vi "Topo & GridSpectr_DriftCorrection_v7.vi"(6 "Internal use":string, 7 "Grid param":T2 {"height (m)" format="%#_6p"; "width (m)" format="%#_6p"; "center Y (m)" format="%#_6p"; "center X (m)" format="%#_6p"}, 8 "Error in (no error)":errorcluster, 9 "Points Y/Index Y":i32, 10 "Points X/Index X":i32, 11 "Method":enum16{"init", "run", "end"}(ring)=enum."end") -> (0 "Error out":errorcluster)   [LabVIEW 2014]
doc: "Example of a measurement VI to be used in the \"Experiments on a Grid\" tool as external VI.\n\nThis example measure the topography and spectroscopy data. The spectroscopy measurements are taken on a subgrid. The data are saved to a sxm and a binary file.\n\n- Nanonis Programming Interface -"
uses:
  <userlib>/Nanonis Prog Interface V5/Nanonis Prog Interface.lvlib
panel:
  in  "max applied Drift Correction":i32=20 min=1 max=100 step=1 format="%.0p"
  in  "Correlate":u16(ring) items=["first Frame", "successive Frames"]
  out "Topo Images taken":i32=14
  in  "Increment":i32=16
  in  "Threshold":i32=3 min=1 step=1
  in  "tip Speed (m/s)":sgl=1e-08 format="%.2p"
  in  "Drift Correction 2":T1
  out "X drift":i32
  out "Y drift":i32
  out "Last Drift detected":i32=40
  in  "MaxImagesBack":i32=40
  in  "Channel index (0-23)":u8=14
  in  "File name":string="single_mol_shortSTS"
  in  "STS Current":dbl=9.999999717180685e-10 format="%#_6p"
  in  "Imaging Current":dbl=5.00000006675716e-11 format="%#_6p"
  in  "zdrift \nDuration (s)":dbl
  in  "Correct z drift":bool
  out "Status":string="finishing"
  in  "Drift correction Pixels":i32=256 caption="Topo Pixels"
  out "Y Offset":dbl format="%#_6p"
  out "X Offset":dbl format="%#_6p"
  out "Points taken":dbl=14.0
  in  "Drift Correction every":i32=16
  in  "Y subgrid spacing":u16=1
  in  "X subgrid spacing":u16=1
  # "GRID points"
  # "Increase this if no Drift was detected for \na certain number of images"
  # "images back"
  # "% of image size"
  # "RUN smart tilt before starting the GRID"
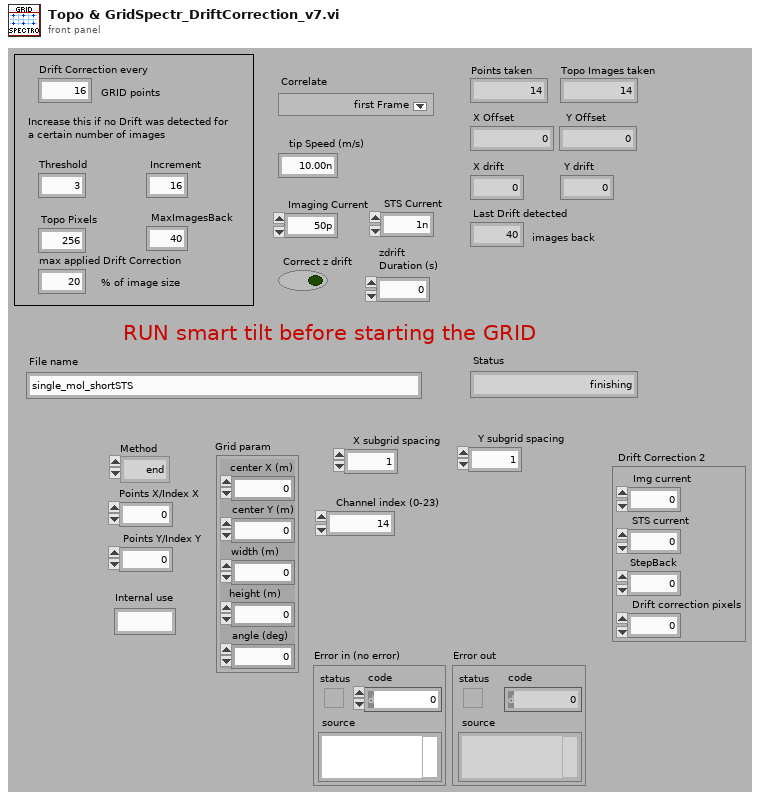
[diagram p1: front panel]
types:
  T1 = cluster{"Img current":dbl, "STS current":dbl, "StepBack":dbl, "Drift correction pixels":dbl}
  T2 = cluster{"center X (m)":sgl, "center Y (m)":sgl, "width (m)":sgl, "height (m)":sgl, "angle (deg)":sgl}
  T3 = cluster{"center X":sgl, "center Y":sgl, "angle":sgl, "width":sgl, "height":sgl, "# pixels":i32, "# lines":i32}
  T4 = cluster{"Name":string, "Calibration":sgl, "Offset":sgl, "Channel index":i32}[]
  T5 = cluster{"up/down":bool, "time/line":sgl, "start time":timestamp, "end time":timestamp}
  T6 = cluster{"Z averaging time (s)":sgl, "Z offset (m)":sgl, "Initial settling time (s)":sgl}
  T7 = cluster{"Max. slew rate (V/s)":sgl, "Settling time (s)":sgl, "Integration time (s)":sgl}
  T8 = cluster{"End settling time (s)":sgl, "Z control time (s)":sgl}
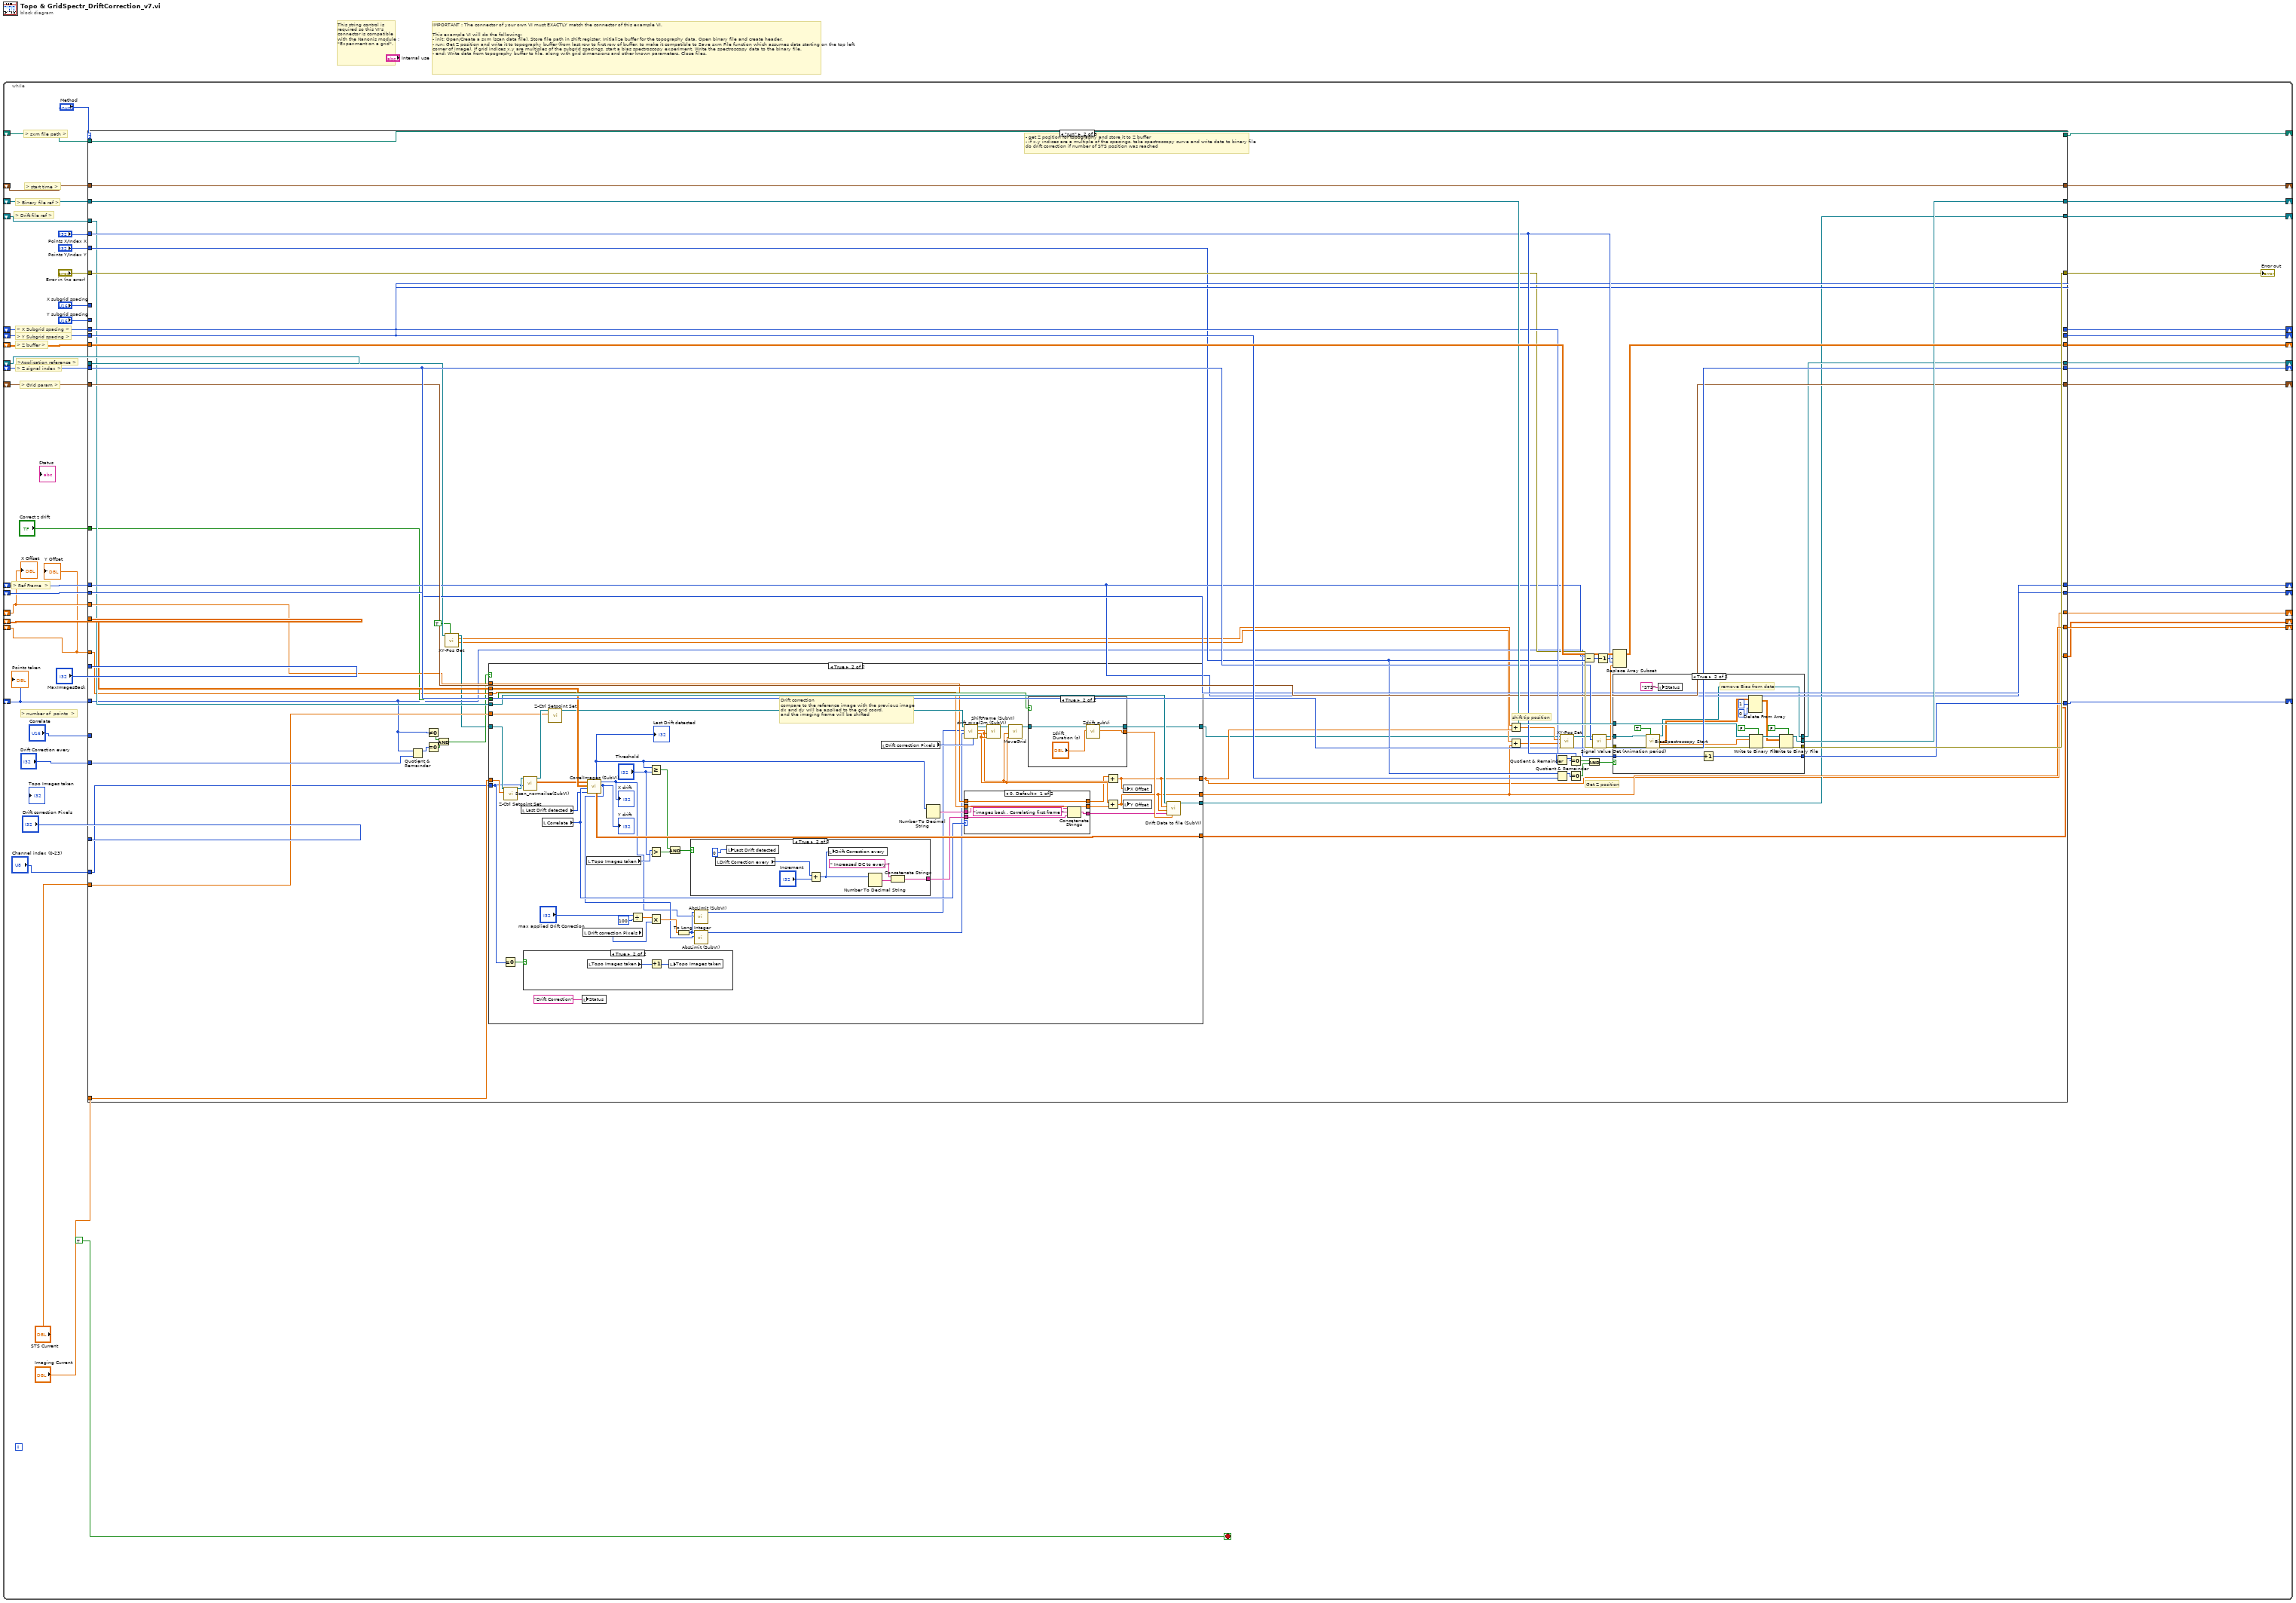
[diagram p0: block diagram]
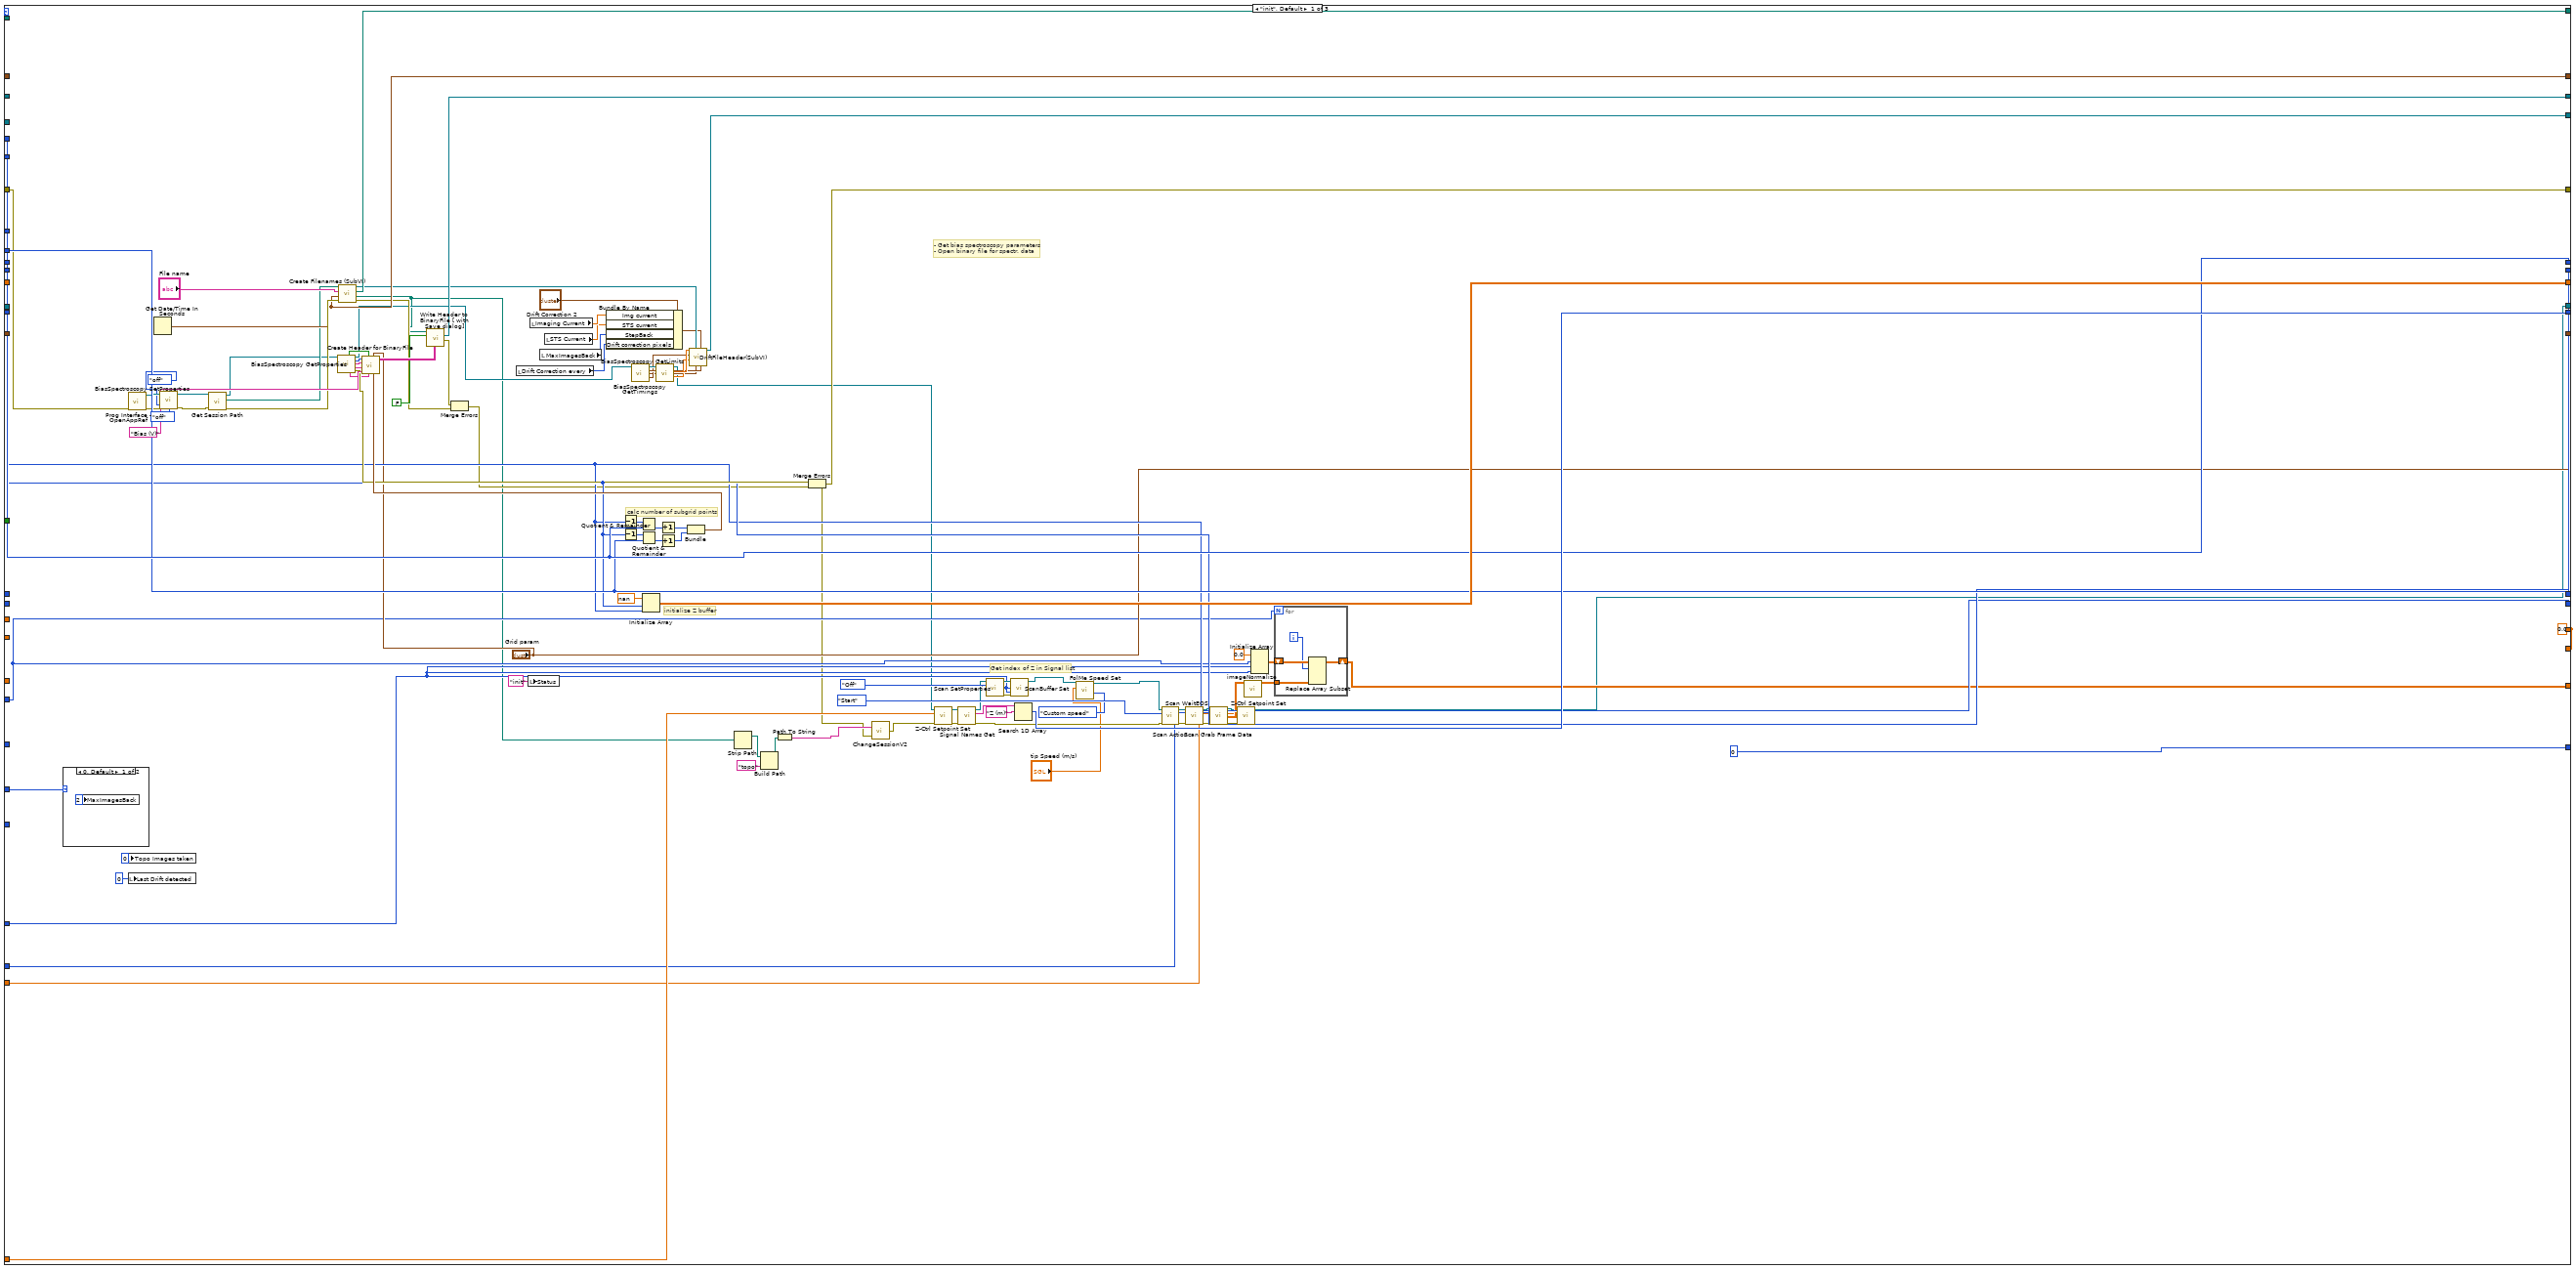
[diagram p2: hidden frame]
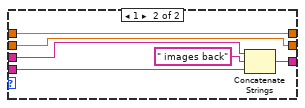
[diagram p5: hidden frame]
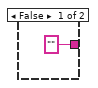
[diagram p7: hidden frame]
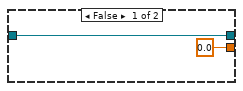
[diagram p8: hidden frame]
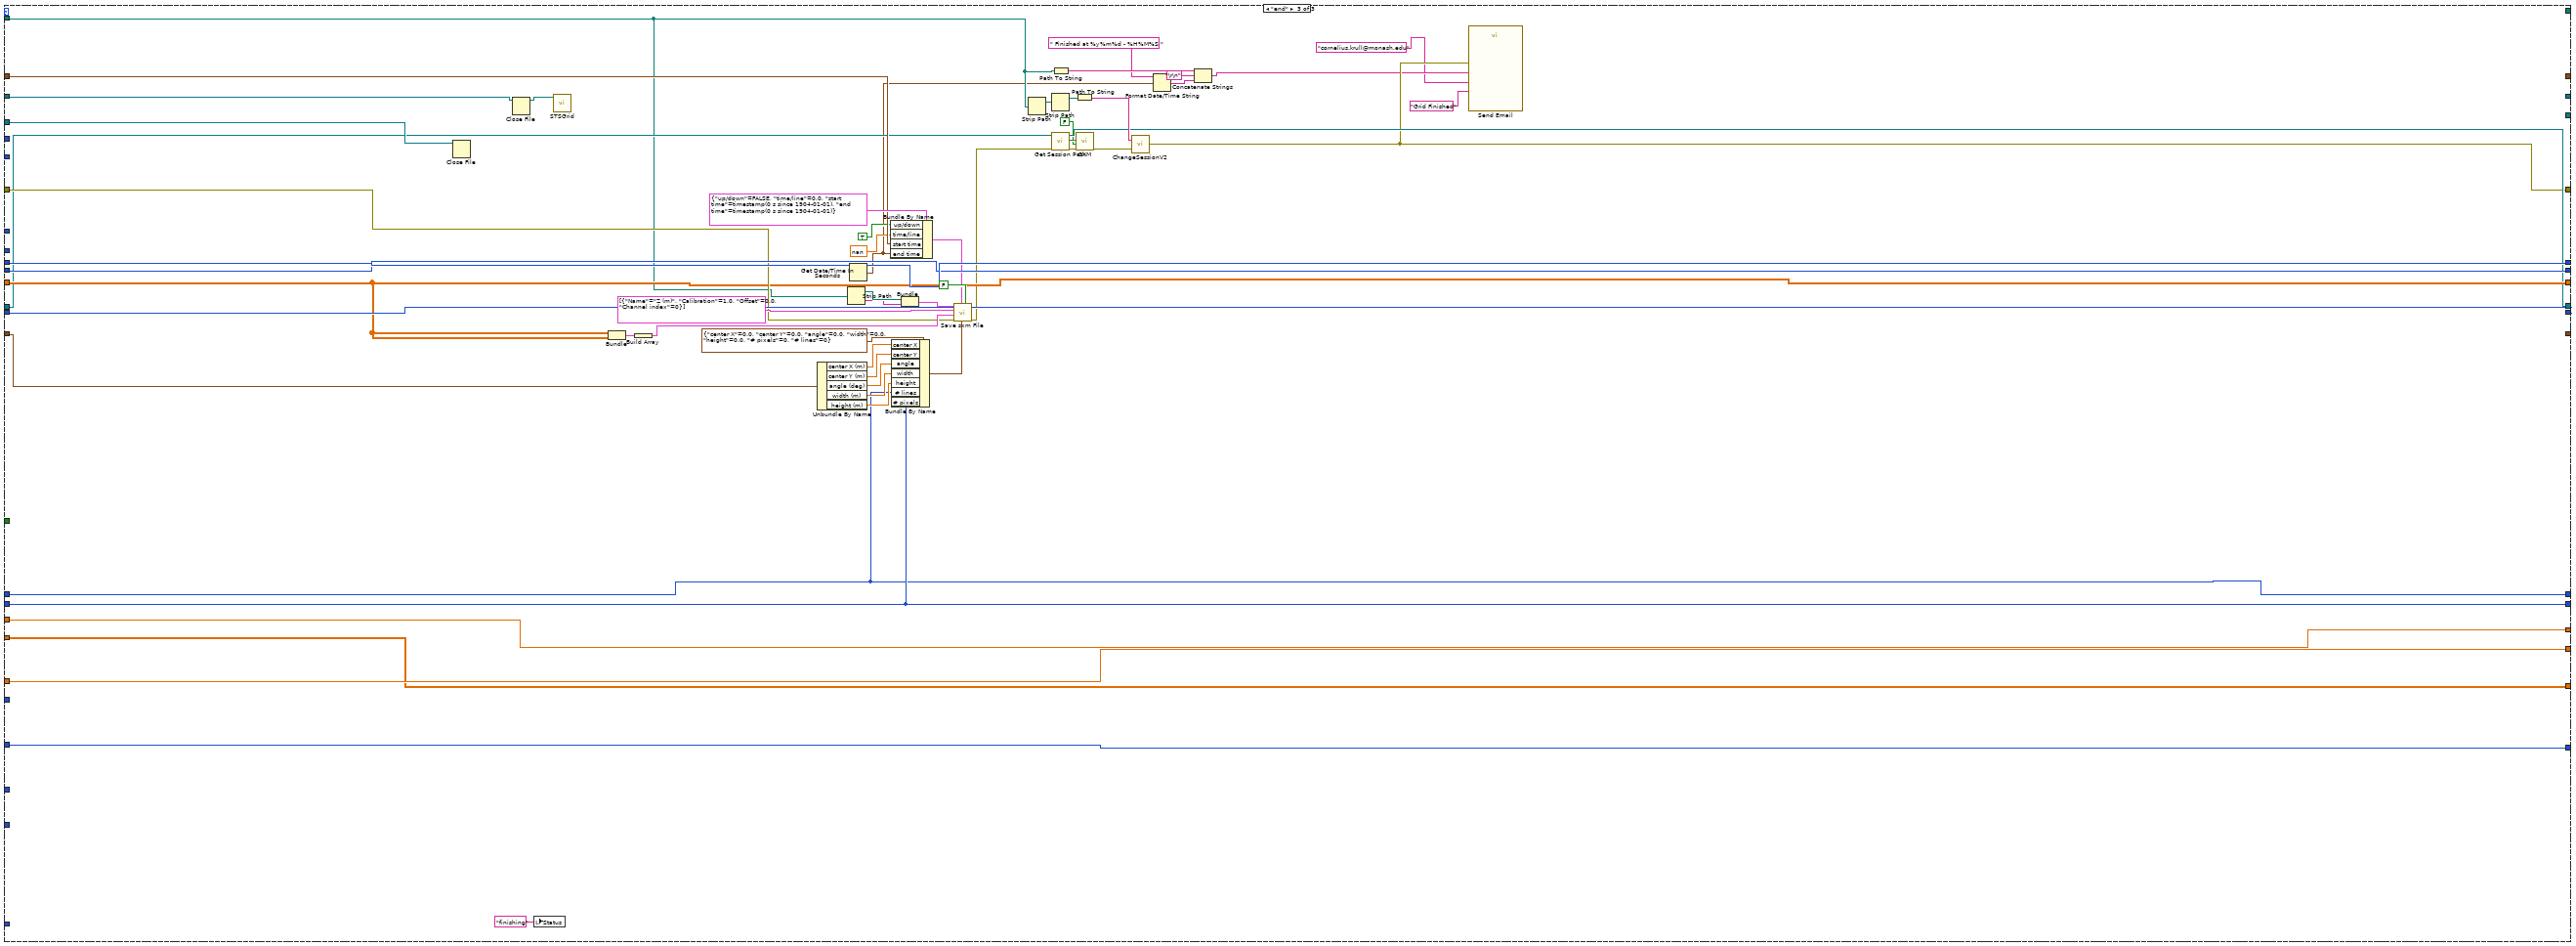
[diagram p10: hidden frame]
diagram:
  # "This string control is required so this VI's connector is compatible with the Nanonis module : \"Experiment on a grid\"."
  # "IMPORTANT : The connector of your own VI must EXACTLY match the connector of this example VI.\n\nThis example VI will do the following:\n- init: Open/Create a sxm (scan data file). Store file path in shift register. Initialize buffer for the topography data. Open binary file and create header.\n- run: Get Z position and write it to topography buffer (from last row to first row of buffer, to make it compatible to Save sxm File function which assumes data starting on the top left corner of image). If grid indices x,y are multiples of the subgrid spacings, start a bias spectroscopy experiment. Write the spectroscopy data to the binary file.\n- end: Write data from topography buffer to file, along with grid dimensions and other known parameters. Close files."
  n1 = while {
    shift-right: [w23] -> _
    shift-left: _ -> [w46]
    shift-right: [w41] -> _
    shift-left: _ -> [w40]
    shift-right: [w38] -> _
    shift-left: _ -> [w39]
    shift-right: [w37] -> _
    shift-left: _ -> [w36]
    shift-right: [w30] -> _
    shift-left: _ -> [w32]
    shift-right: [w31] -> _
    shift-left: _ -> [w33]
    shift-right: [w29] -> _
    shift-left: _ -> [w28]
    shift-right: [w27] -> _
    shift-left: _ -> [w26]
    shift-right: [w25] -> _
    shift-left: _ -> [w24]
    shift-right: [w22] -> _
    shift-left: _ -> [w21]
    shift-right: [w20] -> _
    shift-left: _ -> [w19]
    shift-right: [w18] -> _
    shift-left: _ -> [w11]
    shift-right: [w17] -> _
    shift-left: _ -> [w10]
    shift-right: [w16] -> _
    shift-left: _ -> [w13]
    shift-right: [w15] -> _
    shift-left: _ -> [w12]
    shift-right: [w8] -> _
    shift-left: _ -> [w7]
    stop <- TRUE stop-if-true
    # "> Drift file ref >"
    # "> number of  points  >"
    # "> Ref Frame  >"
    # "> Grid param >"
    # "> start time >"
    # ">Application reference >"
    # "> Y Subgrid spacing >"
    # "> X Subgrid spacing >"
    # "> Z signal index >"
    # "> Binary file ref >"
    # "> Z buffer >"
    # "> sxm file path >"
    n2 = case shown="\"run\"" "Method" {
      tunnel: [w99 w209 _] -> w23
      tunnel: w46 -> [_ w209 w325]
      tunnel: "Error in (no error)" -> [w101 w195 w357]
      tunnel: [w61 w208 w326] -> w44
      tunnel: "Points X/Index X" -> [w125 w203 _]
      tunnel: "Points Y/Index Y" -> [w126 w187 _]
      tunnel: [w149 w206 w346] -> w41
      tunnel: w40 -> [_ w207 w346]
      tunnel: w39 -> [_ w205 w339]
      tunnel: [w141 w204 _] -> w38
      tunnel: [w139 w193 w371] -> w37
      tunnel: w36 -> [_ w193 w371]
      tunnel: "X subgrid spacing" -> [w138 _ _]
      tunnel: "Y subgrid spacing" -> [w137 _ _]
      tunnel: w33 -> [_ w197 w370]
      tunnel: w32 -> [_ w196 w369]
      tunnel: [w138 w197 w370] -> w31
      tunnel: [w137 w196 w369] -> w30
      tunnel: [w72 w179 w331] -> w29
      tunnel: w28 -> [_ w160 w332]
      tunnel: ["Grid param" w190 _] -> w27
      tunnel: w26 -> [_ w190 w356]
      tunnel: [w98 w191 _] -> w25
      tunnel: w24 -> [_ w191 w364]
      tunnel: [w126 w188 w347] -> w22
      tunnel: w21 -> [_ w188 w347]
      tunnel: [w125 w189 w348] -> w20
      tunnel: w19 -> [_ w189 w348]
      tunnel: [w116 w169 w345] -> w18
      tunnel: [w116 w174 w343] -> w17
      tunnel: [w93 w166 w340] -> w16
      tunnel: [0 w184 w344] -> w15
      tunnel: w12 -> [_ w163 w344]
      tunnel: "Drift Correction every" -> [_ w182 _]
      tunnel: w13 -> [_ w173 w340]
      tunnel: w11 -> [_ w180 w345]
      tunnel: w10 -> [_ w164 w343]
      tunnel: "Drift correction Pixels" -> [w92 _ _]
      tunnel: [w88 w171 _] -> w8
      tunnel: w7 -> [_ w172 w341]
      tunnel: "Correct z drift" -> [_ w170 _]
      tunnel: "Imaging Current" -> [w107 w168 _]
      tunnel: "STS Current" -> [w103 w167 _]
      tunnel: "Channel index (0-23)" -> [w96 w165 _]
      tunnel: "MaxImagesBack" -> [w91 _ _]
      tunnel: "Correlate" -> [w52 _ _]
      frame "init", Default {
        w116 = 0.0
        # "- Get bias spectroscopy parameters\n- Open binary file for spectr. data"
        # "initialize Z buffer"
        # "calc number of subgrid points"
        # "Get index of Z in Signal list"
        n3 = case shown="0, Default" w52 {
          frame 0, Default {
            n4 = local write "MaxImagesBack"(2 ("StepsBack")) -> ()
          }
          frame 1 {
          }
        }
        n5 = local write "Topo Images taken"(0 ("Images taken")) -> ()
        n6 = call <userlib>:"Prog Interface - OpenAppRef.vi"("Error in (no error)"=w101) -> ("Error out"=w59:errorcluster, "Application reference"=w102:refnum<vi>)  [unwired: 5 in]
        n7 = local write "Last Drift detected"(0 ("Last Drift detected")) -> ()
        n8 = Get Date/Time In Seconds() -> (seconds since 1Jan1904=w98:timestamp)
        n9 = call <userlib>:"BiasSpectroscopy SetProperties.vi"("Application ref in"=w102, "Autosave (no change)"=enum16{"no change", "on", "off"}."off", "Error in (no error)"=w59, "Save dialog"=enum16{"no change", "on", "off"}."off") -> ("Application ref out"=w55:refnum<vi>, "Error out"=w54:errorcluster)  [unwired: 10 in]
        n10 = call <userlib>:"Get Session Path.vi"("error in (no error)"=w54, "Application ref in"=w55) -> ("error out"=w100:errorcluster, "Session path"=w67:path, "Application ref out"=w56:refnum<vi>)  [unwired: 7 in]
        n11 = call <userlib>:"BiasSpectroscopy GetProperties.vi"("Application ref in"=w56) -> ("Backward sweep"=w145:bool, "Application ref out"=w71:refnum<vi>, "Number of points"=w128:i32, "Channels"=w127:string[], "Parameters"=w143:string[], "Fixed parameters"=w130:string[], "Error out"=w142:errorcluster)  [unwired: 6 in, 2 out]
        n12 = call "Create Filenames (SubVI).vi"("error in (no error)"=w100, "seconds since 1Jan1904"=w98, "File name"="File name", "Session path"=w67) -> ("error out"=w73:errorcluster, "binFilePath"=w63:path, "topoFilePath"=w99:path, "Drift File out"=w89:refnum<file>)  [unwired: 4 in]
        n13 = local read "Drift Correction every"() -> (w83:i32)
        n14 = local write "Status"("init" ("Status")) -> ()
        n15 = local read "Imaging Current"() -> (w85:dbl)
        n16 = local read "MaxImagesBack"() -> (w82:i32)
        n17 = local read "STS Current"() -> (w84:dbl)
        n18 = Bundle By Name(cluster="Drift Correction 2", "Img current"=w85, "STS current"=w84, "StepBack"=w82, "Drift correction pixels"=w83) -> (w86:T1)
        n19 = Decrement(x=w125) -> (x-1=w136:i32)
        n20 = Decrement(x=w126) -> (x-1=w135:i32)
        n21 = call <userlib>:"BiasSpectroscopy GetTimings.vi"("Application ref in"=w71) -> ("Application ref out"=w81:refnum<vi>, "Initialization"=w78:T6, "Sweep Timing"=w76:T7, "End of Sweep"=w77:T8)  [unwired: 10 in, 1 out]
        n22 = Quotient & Remainder(x=w136, y=w138) -> (floor(x/y)=w134:i32)  [unwired: 1 out]
        n23 = Quotient & Remainder(x=w135, y=w137) -> (floor(x/y)=w133:i32)  [unwired: 1 out]
        n24 = Initialize Array(sgl nan ("element"), w126, w125) -> (w149:sgl[][])
        n25 = call <userlib>:"BiasSpectroscopy GetLimits.vi"("Application ref in"=w81) -> ("End value (V)"=w79:sgl, "Start value (V)"=w80:sgl, "Application ref out"=w49:refnum<vi>)  [unwired: 5 in, 1 out]
        n26 = Increment(x=w134) -> (x+1=w132:i32)
        n27 = Increment(x=w133) -> (x+1=w131:i32)
        n28 = Bundle(w132, w131) -> (w144:cluster{i32, i32})  [unwired: 1 in]
        n29 = call <userlib>:"Create Header for BinaryFile.vi"("Grid points"=w144, "Grid param"="Grid param", "Fixed parameters"=w130, "Backward sweep"=w145, "Sweep signal"="Bias (V)" ("Sweep Signal"), "Parameters"=w143, "Channels"=w127, "Points per sweep"=w128) -> ("Header (fixed attributes)"=w147:string[][])  [unwired: 3 in]
        n30 = call <userlib>:"Write Header to BinaryFile [ with Save dialog].vi"("Fixed Attributes"=w147, "Show Dialog? (T)"=FALSE, "Filename"=w63) -> ("Error out"=w74:errorcluster, "File ref"=w141:refnum<file>)  [unwired: 5 in, 2 out]
        n31 = Merge Errors(w74, w73) -> (w75:errorcluster)
        n32 = call "DriftFileHeader(SubVI).vi"("Initialization"=w78, "Drift Correction"=w86, "Sweep Timing"=w76, "Byte Stream File in"=w89, "End value (V)"=w79, "End of Sweep"=w77, "Start value (V)"=w80) -> ("Byte Stream File out"=w88:refnum<file>)  [unwired: 4 in]
        n33 = Strip Path(path=w63) -> (stripped path=w66:path)  [unwired: 1 out]
        n34 = Build Path(base path=w66, name or relative path="topo") -> (appended path=w64:path)
        n35 = Path To String(path=w64) -> (string=w62:string)
        n36 = Merge Errors(w142, w75) -> (w61:errorcluster)
        n37 = call "ChangeSessionV2.vi"("error in (no error)"=w61, "Session"=w62) -> ("error out"=w60:errorcluster)
        n38 = call <userlib>:"Z-Ctrl Setpoint Set.vi"("error in (no error)"=w60, "Z Controller setpoint"=w107, "Application ref in"=w49) -> ("error out"=w106:errorcluster, "Application ref out"=w108:refnum<vi>)  [unwired: 7 in]
        n39 = call <userlib>:"Signal Names Get.vi"("error in (no error)"=w106, "Application ref in"=w108) -> ("error out"=w117:errorcluster, "Signals Names"=w129:string[], "Application ref out"=w112:refnum<vi>)  [unwired: 5 in]
        n40 = call <userlib>:"Scan SetProperties.vi"("Application ref in"=w112, "Continuous scan"=enum16{"No change", "On", "Off"}."Off") -> ("Application ref out"=w114:refnum<vi>, "Error out"=w113:errorcluster)  [unwired: 12 in]
        n41 = call <userlib>:"ScanBuffer Set.vi"("Application ref in"=w114, "Pixels"=w92, "Lines"=w92, "error in (no error)"=w113) -> ("Application ref out"=w50:refnum<vi>)  [unwired: 10 in, 1 out]
        n42 = Search 1D Array(1D array=w129, element="Z (m)") -> (index of element=w139:i32)  [unwired: 1 in]
        n43 = call <userlib>:"FolMe Speed Set.vi"("Speed Setting (Custom)"=enum32{"Scan speed", "Custom speed"}."Custom speed", "Speed (m/s)"="tip Speed (m/s)", "Application ref in"=w50) -> ("Application ref out"=w70:refnum<vi>)  [unwired: 5 in, 1 out]
        n44 = call <userlib>:"Scan Action.vi"("error in (no error)"=w117, "Scan action (Start)"=enum16{"Start", "Stop", "Pause", "Resume"}."Start", "Application ref in"=w70) -> ("error out"=w123:errorcluster, "Application ref out"=w122:refnum<vi>)  [unwired: 6 in]
        n45 = call <userlib>:"Scan WaitEOS.vi"("error in (no error)"=w123, "Application ref in"=w122) -> ("error out"=w120:errorcluster, "Application ref out"=w121:refnum<vi>)  [unwired: 5 in, 2 out]
        n46 = call <userlib>:"Scan Grab Frame Data.vi"("Application ref in"=w121, "Channel index (0-23)"=w96, "error in (no error)"=w120) -> ("Application ref out"=w105:refnum<vi>, "Scan frame data"=w109:sgl[][], "error out"=w104:errorcluster)  [unwired: 8 in, 2 out]
        n47 = call <userlib>:"Z-Ctrl Setpoint Set.vi"("error in (no error)"=w104, "Z Controller setpoint"=w103, "Application ref in"=w105) -> ("Application ref out"=w72:refnum<vi>)  [unwired: 7 in, 1 out]
        n48 = call "imageNormalize.vi"("Data"=w109) -> ("Array"=w90:dbl[][])  [unwired: 10 in]
        n49 = Initialize Array(0.0 ("element"), w91, w92, w92) -> (w94:dbl[][][])
        n50 = for {
          N: w91 -> [_]
          tunnel: w90 -> [w153]
          shift-right: [w152] -> w93
          shift-left: w94 -> [w154]
          i -> [w151]
          n51 = Replace Array Subset(array=w154, new element=w153, index (dim 0)=w151) -> (w152:dbl[][][])  [unwired: 2 in]
        }
      }
      frame "run" {
        # "shift tip position"
        # "Get Z position"
        # "- get Z position for topography and store it to Z buffer\n- if x,y indices are a multiple of the spacings, take spectroscopy curve and write data to binary file\ndo drift correction if number of STS position was reached"
        n52 = Quotient & Remainder(x=w163, y=w182) -> (x-y*floor(x/y)=w183:i32)  [unwired: 1 out]
        n53 = Not Equal To 0?(x=w163) -> (x != 0?=w161:bool)
        n54 = Equal To 0?(x=w183) -> (x = 0?=w181:bool)
        n55 = And(x=w161, y=w181) -> (x .and. y?=w162:bool)
        n56 = call <userlib>:"XY-Pos Get.vi"("Wait for newest data (F=False)"=TRUE, "Application ref in"=w160) -> ("Y (m)"=w156:sgl, "X (m)"=w157:sgl, "Application ref out"=w159:refnum<vi>)  [unwired: 5 in, 1 out]
        n57 = case shown="True" w162 {
          tunnel: w159 -> [w214 w256]
          tunnel: [w214 w260] -> w155
          tunnel: w173 -> [w211 w251]
          tunnel: [w213 w258] -> w169
          tunnel: [w212 w257] -> w174
          tunnel: w180 -> [w213 w230]
          tunnel: w164 -> [w212 w228]
          tunnel: [w211 w247] -> w166
          tunnel: w172 -> [w210 w263]
          tunnel: [w210 w262] -> w171
          tunnel: w170 -> [_ w259]
          tunnel: w168 -> [_ w255]
          tunnel: w167 -> [_ w253]
          tunnel: w165 -> [_ w234]
          frame False {
          }
          frame True {
            # "Drift correction \ncompare to the reference image with the previous image \ndx and dy will be applied to the grid coord, \nand the imaging frame will be shifted"
            n58 = Greater Or Equal To 0?(x=w234) -> (x >= 0?=w233:bool)
            n59 = call <userlib>:"Z-Ctrl Setpoint Set.vi"("Z Controller setpoint"=w255, "Application ref in"=w256) -> ("Application ref out"=w252:refnum<vi>)  [unwired: 8 in, 1 out]
            n60 = local read "Last Drift detected"() -> (w225:i32)
            n61 = call "Scan_normailze(SubVI).vi"("Channel index (0-23)"=w234, "Application in"=w252) -> ("Array"=w248:dbl[][], "Application out"=w254:refnum<vi>)  [unwired: 7 in, 1 out]
            n62 = case shown="True" w233 {
              frame False {
              }
              frame True {
                n63 = local read "Topo Images taken"() -> (w278:i32)
                n64 = Increment(x=w278) -> (x+1=w277:i32)
                n65 = local write "Topo Images taken"(w277) -> ()
              }
            }
            n66 = local read "Correlate"() -> (w231:u16)
            n67 = call <userlib>:"Z-Ctrl Setpoint Set.vi"("Z Controller setpoint"=w253, "Application ref in"=w254) -> ("Application ref out"=w243:refnum<vi>)  [unwired: 8 in, 1 out]
            n68 = local write "Status"("Drift Correction" ("Status")) -> ()
            n69 = local read "Drift correction Pixels"() -> (w222:i32)
            n70 = local read "Topo Images taken"() -> (w236:i32)
            n71 = call "CorrelImages (SubVI).vi"("last drift detected"=w225, "Correlate"=w231, "Ref Array"=w251, "New Image"=w248) -> ("Y drift"=w219:i32, "X drift"=w216:i32, "Ref Array out"=w247:dbl[][][], "Queue Steps"=w232:i32)  [unwired: 4 in]
            "X drift" <- w216
            "Y drift" <- w219
            "Last Drift detected" <- w232
            n72 = Divide(x="max applied Drift Correction", y=100) -> (x/y=w221:dbl)
            n73 = Greater Or Equal?(x=w232, y="Threshold") -> (x >= y?=w238:bool)
            n74 = Greater?(x=w236, y="Threshold") -> (0:w235:bool)
            n75 = Multiply(x=w221, y=w222) -> (x*y=w223:dbl)
            n76 = And(x=w238, y=w235) -> (x .and. y?=w237:bool)
            n77 = To Long Integer(number=w223) -> (32bit integer=w215:i32)
            n78 = case shown="True" w237 {
              tunnel: ["" w282] -> w239
              frame False {
              }
              frame True {
                n79 = local read "Drift Correction every"() -> (w281:i32)
                n80 = local write "Last Drift detected"(0 ("Last Drift detected")) -> ()
                n81 = Add(x=w281, y="Increment") -> (x+y=w285:i32)
                n82 = local write "Drift Correction every"(w285) -> ()
                n83 = Number To Decimal String(number=w285) -> (decimal integer string=w284:string)  [unwired: 1 in]
                n84 = Concatenate Strings(" Increased DC to every " ("string"), w284) -> (w282:string)
              }
            }
            n85 = call "AbsLimit (SubVI).vi"("in"=w216, "Abslimt"=w215) -> ("Numeric out"=w218:i32)  [unwired: 9 in]
            n86 = call "AbsLimit (SubVI).vi"("in"=w219, "Abslimt"=w215) -> ("Numeric out"=w217:i32)  [unwired: 9 in]
            n87 = local read "Drift correction Pixels"() -> (w244:i32)
            n88 = Number To Decimal String(number=w232) -> (decimal integer string=w250:string)  [unwired: 1 in]
            n89 = call "drift_pixel2m (SubVI).vi"("Application in"=w243, "X drift"=w218, "Y drift"=w217, "Drift correction Pixels"=w244) -> ("Application out"=w242:refnum<vi>, "x drift"=w240:sgl, "y drift"=w241:sgl)  [unwired: 2 in, 1 out]
            n90 = case shown="0, Default" w231 {
              tunnel: w250 -> [w265 w276]
              tunnel: [w270 w275] -> w249
              tunnel: w239 -> [w268 w273]
              tunnel: w230 -> [w266 w272]
              tunnel: [w266 w272] -> w229
              tunnel: w228 -> [w267 w271]
              tunnel: [w267 w271] -> w227
              frame 0, Default {
                n91 = Concatenate Strings(w265, "images back , Correlating first frame " ("string"), w268) -> (w270:string)
              }
              frame 1 {
                n92 = Concatenate Strings(w276, " images back" ("string"), w273) -> (w275:string)
              }
            }
            n93 = call "ShiftFrame (SubVI).vi"("Y shift"=w241, "X shift"=w240, "Application in"=w242) -> ("Application out"=w246:refnum<vi>)  [unwired: 8 in]
            n94 = call "MoveGrid.vi"("y"=w241, "x"=w240, "Application ref in"=w246) -> ("Application ref out"=w245:refnum<vi>)  [unwired: 7 in, 1 out]
            n95 = case shown="True" w259 {
              tunnel: [0.0 ("z drift") w292] -> w261
              tunnel: w245 -> [w287 w291]
              tunnel: [w287 w290] -> w260
              frame False {
              }
              frame True {
                n96 = call "Zdrift_subVi.vi"("Duration"="zdrift \nDuration (s)", "Application in"=w291) -> ("z drift"=w292:dbl, "Application out"=w290:refnum<vi>)  [unwired: 7 in, 1 out]
              }
            }
            n97 = Add(x=w229, y=w240) -> (x+y=w258:dbl)
            n98 = Add(x=w241, y=w227) -> (x+y=w257:dbl)
            n99 = local write "X Offset"(w258) -> ()
            n100 = local write "Y Offset"(w257) -> ()
            n101 = call "Drift Data to file (SubVI).vi"("z drift"=w261, "Comment"=w249, "y Drift"=w257, "X drift"=w258, "Byte Stream File in"=w263) -> ("Byte Stream File out"=w262:refnum<file>)  [unwired: 6 in]
          }
        }
        n102 = Add(x=w157, y=w169) -> (x+y=w176:dbl)
        n103 = Add(x=w156, y=w174) -> (x+y=w175:dbl)
        n104 = Quotient & Remainder(x=w203, y=w197) -> (x-y*floor(x/y)=w202:i32)  [unwired: 1 out]
        n105 = Quotient & Remainder(x=w187, y=w196) -> (x-y*floor(x/y)=w201:i32)  [unwired: 1 out]
        n106 = call <userlib>:"XY-Pos Set.vi"("Y (m)"=w175, "X (m)"=w176, "Application ref in"=w155) -> ("Application ref out"=w177:refnum<vi>)  [unwired: 5 in, 1 out]
        n107 = Equal To 0?(x=w202) -> (x = 0?=w200:bool)
        n108 = Equal To 0?(x=w201) -> (x = 0?=w199:bool)
        n109 = Subtract(x=w188, y=w187) -> (x-y=w186:i32)
        n110 = And(x=w200, y=w199) -> (x .and. y?=w198:bool)
        n111 = call <userlib>:"Signal Value Get (Animation period).vi"("error in (no error)"=w195, "Signal index (0-47)"=w193, "Application ref in"=w177) -> ("error out"=w194:errorcluster, "Signal value"=w192:sgl, "Application ref out"=w178:refnum<vi>)  [unwired: 5 in]
        n112 = Decrement(x=w186) -> (x-1=w185:i32)
        n113 = Replace Array Subset(array=w207, new element=w192, index (row)=w185, index (col)=w203) -> (w206:sgl[][])
        n114 = case shown="True" w198 {
          tunnel: [w295 w300] -> w208
          tunnel: w205 -> [w296 w316]
          tunnel: [w296 w314] -> w204
          tunnel: w194 -> [w295 w313]
          tunnel: w178 -> [w294 w305]
          tunnel: [w294 w304] -> w179
          tunnel: [w293 w298] -> w184
          tunnel: w163 -> [w293 w299]
          frame False {
            # "Point indices aren't multiple of subgrid spacing\n=> no spectroscopy at this point"
          }
          frame True {
            # "remove Bias from data"
            n115 = call <userlib>:"BiasSpectroscopy Start.vi"("Application ref in"=w305, "Get data (F)"=TRUE ("Get Data (F)"), "Error in (no error)"=w313) -> ("Application ref out"=w304:refnum<vi>, "Data"=w312:sgl[][], "Parameters"=w311:sgl[], "Error out"=w302:errorcluster)  [unwired: 8 in, 1 out]
            n116 = local write "Status"("STS" ("Status")) -> ()
            n117 = Increment(x=w299) -> (x+1=w298:i32)
            n118 = Delete From Array(array=w312, length=1, index (row)=0 ("index")) -> (array with subset deleted=w310:sgl[][])  [unwired: 1 in, 1 out]
            n119 = Write to Binary File(file (use dialog)=w316, data=w311, error in=w302, 5:FALSE ("prepend array or string size? (T)")) -> (refnum out=w315:refnum<file>, error out=w301:errorcluster)  [unwired: 2 in, 1 out]
            n120 = Write to Binary File(file (use dialog)=w315, data=w310, error in=w301, 5:FALSE ("prepend array or string size? (T)")) -> (refnum out=w314:refnum<file>, error out=w300:errorcluster)  [unwired: 2 in, 1 out]
          }
        }
      }
      frame "end" {
        n121 = Close File(refnum=w341) -> ()  [unwired: 1 in, 2 out]
        n122 = Close File(refnum=w339) -> (path=w338:path)  [unwired: 1 in, 1 out]
        n123 = local write "Status"("finishing" ("Status")) -> ()
        n124 = call "STSGrid.vi"("Binary Spectroscopy File"=w338) -> ()  [unwired: 11 in]
        n125 = Bundle(w346, w346) -> (w368:cluster{sgl[][], sgl[][]})  [unwired: 1 in]
        n126 = Build Array(w368) -> (w367:cluster{sgl[][], sgl[][]}[])
        n127 = Unbundle By Name(w356) -> ("center X (m)"=w354:sgl, "center Y (m)"=w353:sgl, "angle (deg)"=w352:sgl, "width (m)"=w351:sgl, "height (m)"=w350:sgl)
        n128 = Strip Path(path=w325) -> (stripped path=w360:path, name=w359:string)
        n129 = Get Date/Time In Seconds() -> (seconds since 1Jan1904=w320:timestamp)
        n130 = Bundle By Name(cluster=T5 {"up/down"=FALSE, "time/line"=0.0, "start time"=timestamp(0 s since 1904-01-01), "end time"=timestamp(0 s since 1904-01-01)} ("Scan param"), "up/down"=TRUE, "time/line"=sgl nan ("input 7"), "start time"=w364, "end time"=w320) -> (w363:T5)
        n131 = Bundle By Name(cluster=T3 {"center X"=0.0, "center Y"=0.0, "angle"=0.0, "width"=0.0, "height"=0.0, "# pixels"=0, "# lines"=0} ("Scanfield"), "center X"=w354, "center Y"=w353, "angle"=w352, "width"=w351, "height"=w350, "# lines"=w347, "# pixels"=w348) -> (w349:T3)
        n132 = Bundle("stripped path"=w360, "name"=w359) -> (w358:cluster{"stripped path":path, "name":string})  [unwired: 1 in]
        n133 = call <userlib>:"Save sxm File.vi"("Auto file naming? (T)"=FALSE, "Scanfield"=w349, "Scan param"=w363, "error in (no error)"=w357, "Channels data"=w367, "Channels config"=T4 [{"Name"="Z (m)", "Calibration"=1.0, "Offset"=0.0, "Channel index"=0}], "Filename control"=w358) -> ("error out"=w333:errorcluster)  [unwired: 2 in, 2 out]
        n134 = Strip Path(path=w325) -> (stripped path=w337:path)  [unwired: 1 out]
        n135 = Strip Path(path=w337) -> (stripped path=w336:path)  [unwired: 1 out]
        n136 = call <userlib>:"Get Session Path.vi"("error in (no error)"=w333, "Application ref in"=w332) -> ("error out"=w328:errorcluster, "Session path"=w330:path, "Application ref out"=w331:refnum<vi>)  [unwired: 7 in]
        n137 = Path To String(path=w325) -> (string=w324:string)
        n138 = Path To String(path=w336) -> (string=w334:string)
        n139 = call "SXM.vi"("Path"=w330, "Delete"=FALSE, "error in"=w328) -> ("error out"=w327:errorcluster)  [unwired: 7 in]
        n140 = call "ChangeSessionV2.vi"("error in (no error)"=w327, "Session"=w334) -> ("error out"=w326:errorcluster)
        n141 = Format Date/Time String(time format string (%c)=" Finished at %y%m%d - %H%M%S ", seconds (now)=w320) -> (date/time string=w319:string)  [unwired: 1 in]
        n142 = Concatenate Strings(w324, "\r\n", w319) -> (w322:string)
        n143 = call "Send Email"("error in"=w326, "Message"=w322, "Subject"="Grid Finished", "Recipients"="cornelius.krull@monash.edu") -> ()  [unwired: 7 in, 1 out]
      }
    }
    "Error out" <- w44
    "Points taken" <- w12
    "X Offset" <- w11
    "Y Offset" <- w10
  }
